vi "NML Signal Average.vi"() -> ()   [LabVIEW 2021]
doc: "Averages N cylces of input. Input is syncronized to a square wave output from DAC 1, DAC 0 is the drive of the given amplitude and duty cylce. Dac 1 should be connected to EXT Trigger, (make sure that DAC 1 has an external reference voltage of at least 1 V)\nScott Hannahs, FBNML, Jan 1992"
uses:
  <vilib>/_DAQmxBase/Internals/Properties/WriteProperties/RegenMode.ctl
  <vilib>/_DAQmxBase/Internals/DAQmxBase Create Channel (AO-Voltage-Basic).vi
  <vilib>/_DAQmxBase/Internals/DAQmxBase Timing (Sample Clock).vi
  <vilib>/_DAQmxBase/Internals/Properties/WriteProperties/Set_Write_RegenMode.vi
  <vilib>/_DAQmxBase/Internals/DAQmxBase Write (Analog 2D DBL NChan NSamp).vi
  <vilib>/_DAQmxBase/Internals/DAQmxBase Read (Analog 2D DBL NChan NSamp).vi
panel:
  out "Errors:":string
  out "?":dbl[](graph)
  out "Output Data":sgl[](array[numeric])=[0.032989502, 0.0625, 0.09112549, 0.12008667, 0.14807129, 0.17654419, 0.20431519, 0.23254395, 0.25964355, 0.2871704, 0.3139038, 0.34094238, 0.3671875, 0.39404297, 0.4197998, 0.44604492, 0.47161865, 0.49743652, 0.5225525, 0.5479126, 0.5722656, 0.59713745, 0.6213989, 0.64608765, 0.66989136, 0.6939392, 0.7173462, 0.74108887, 0.76416016, 0.78775024, 0.8104553, 0.8332825, 0.8556824, 0.8781738, 0.8999939, 0.9222717, 0.9437561, 0.9659729, 0.9867554, 1.0085449, 1.0292664, 1.0500183, 1.0709839, 1.0917358, 1.1118164, 1.1324463, 1.1521912, 1.1723633, 1.1917725, 1.2114258, 1.230835, 1.2502136, 1.2690735, 1.2883301, 1.3070068, 1.3257141, 1.3437195, 1.3625793, 1.3806763, 1.3986816, 1.4164429, 1.4342651, 1.4515991, 1.4693909, 1.4862976, 1.5037231, 1.5204773, 1.5375671, 1.5540771, 1.5710144, 1.5870056, 1.6036377, 1.6196594, 1.6356812, 1.6517029, 1.667572, 1.6828003, 1.6987, 1.7136536, 1.7294922, 1.7442322, 1.759552, 1.7741699, 1.7893372, 1.8037415, 1.8181763, 1.8328247, 1.8470154, 1.8611755, 1.8754272, 1.888977, 1.9031067, 1.9164734, 1.9305115, 1.9437256, 1.9572754, 1.9702454, 1.9837036, 1.9964905, 2.0097961, 2.0221863, 2.0352173, 2.047638, 2.0603638, 2.0722046, 2.0852966, 2.097107, 2.109314, 2.1211853, 2.1333008, 2.144867, 2.1571655, 2.1681519, 2.1801147, 2.190979, 2.2028503, 2.2136536, 2.2251282, 2.235962, 2.2472534, 2.2578125, 2.2688293, 2.2792969, 2.2900696, 2.3004456, 2.3112183, 2.3211975, 2.3319702, 2.3417053, 2.3520508, 2.3616333, 2.3719788, 2.3815613, 2.3916016, 2.4009705, 2.4106445, 2.4199219, 2.42984, 2.4389648, 2.4486694, 2.4572144, 2.4668884, 2.4756165, 2.4849548, 2.4935608, 2.502594, 2.5106506, 2.519806, 2.5283508, 2.5372314, 2.5454407, 2.5540466, 2.5621948, 2.5708008, 2.5786438, 2.5872192, 2.5947266, 2.6029663, 2.6105957, 2.618805, 2.6265564, 2.634552, 2.6419373, 2.6497803, 2.6569824, 2.6648865, 2.6722412, 2.679657, 2.686554, 2.694458, 2.7011414, 2.7087708, 2.715271, 2.7225342, 2.729309, 2.7364502, 2.7431946, 2.7503052, 2.7565002, 2.7634583, 2.7698975, 2.7767944, 2.782837, 2.7895813, 2.795929, 2.8024597, 2.8084412, 2.8148193, 2.8210754, 2.82724, 2.8332214, 2.8396606, 2.8454285, 2.8513184, 2.856842, 2.8631287, 2.868866, 2.8746338, 2.8800354, 2.8859863, 2.8912964, 2.8970642, 2.9022217, 2.9082336, 2.913147, 2.9189148, 2.9239807, 2.929596, 2.9346313, 2.940094, 2.9449158, 2.950409, 2.9551697, 2.9606323, 2.965332, 2.9704895, 2.9749756, 2.9799194, 2.9845886, 2.9897766, 2.9943848, 2.9996338, 3.003662, 3.008667, 3.0127563, 3.0178833, 3.0220642, 3.0269165, 3.0310059, 3.0357056, 3.0396423, 3.044403, 3.0485535, 3.0531006, 3.0569763, 3.061432, 3.065277, 3.0694275, 3.0734253, 3.0778198, 3.0814514, 3.085846, 3.0895996, 3.0937195, 3.09729, 3.10141, 3.1050415, 3.1092834, 3.1127625, 3.1166382, 3.1201172, 3.1239624, 3.127411, 3.131256, 3.1345215, 3.1383057, 3.142334, 3.1159668, 3.0895996, 3.0645142, 3.0388184, 3.0143738, 2.9890747, 2.9644775, 2.9400635, 2.9158325, 2.8914185, 2.8678894, 2.8439636, 2.8207703, 2.7972107, 2.774353, 2.7512207, 2.7288208, 2.705841, 2.684021, 2.6614075, 2.639923, 2.6178894, 2.596405, 2.574707, 2.5537415, 2.532318, 2.5117493, 2.4907227, 2.4706726, 2.4499512, 2.4298096, 2.4098816, 2.3901367, 2.3703003, 2.350708, 2.3310852, 2.3123474, 2.292633, 2.274109, 2.255127, 2.236969, 2.2182007, 2.2000122, 2.1818237, 2.1638489, 2.145996, 2.1282654, 2.1105347, 2.0935364, 2.0758057, 2.0591736, 2.041626, 2.025299, 2.0080566, 1.9917297, 1.9750977, 1.959259, 1.9427185, 1.927063, 1.910675, 1.8952637, 1.8792725, 1.8640747, 1.8486328, 1.8333435, 1.8180237, 1.8032837, 1.788269, 1.7736816, 1.7590637, 1.74469, 1.7299194, 1.716095, 1.7011719, 1.6877136, 1.6734314, 1.6602173, 1.6459961, 1.6327515, 1.6190186, 1.6058044, 1.5922852, 1.5796509, 1.5662842, 1.5537109, 1.5403748, 1.5280762, 1.5151672, 1.5027771, 1.4902039, 1.4781799, 1.4660339, 1.4541321, 1.4414673, 1.4299927, 1.4178162, 1.4064636, 1.3948059, 1.3835754, 1.3715515, 1.3607178, 1.348938, 1.3382568, 1.327179, 1.3163452, 1.3050232, 1.2947998, 1.283905, 1.2733765, 1.2626038, 1.2525635, 1.2420654, 1.231842, 1.2216797, 1.2118225, 1.2011414, 1.1916809, 1.1815186, 1.1719971, 1.1622009, 1.152832, 1.1428223, 1.1341858, 1.1242981, 1.1152039, 1.1057434, 1.0970459, 1.0876465, 1.07901, 1.0698547, 1.0611267, 1.052063, 1.0437622, 1.0348816, 1.0266418, 1.0179749, 1.0097351, 1.0010376, 0.9930725, 0.9847412, 0.97680664, 0.96832275, 0.96087646, 0.9525757, 0.9450073, 0.9370117, 0.92941284, 0.9214783, 0.9143677, 0.9063721, 0.89920044, 0.8913269, 0.8841553, 0.876709, 0.86987305, 0.86242676, 0.85549927, 0.84802246, 0.84140015, 0.83432007, 0.8274536, 0.8204651, 0.81411743, 0.80700684, 0.80062866, 0.79367065, 0.78744507, 0.7805481, 0.7746582, 0.76782227, 0.76171875, 0.7552185, 0.74902344, 0.7426758, 0.7367554, 0.7305298, 0.7247925, 0.7187195, 0.71273804, 0.70651245, 0.7012634, 0.6950989, 0.68969727, 0.68362427, 0.67837524, 0.67245483, 0.6670532, 0.6612549, 0.65625, 0.6502075, 0.64541626, 0.63986206, 0.6348877, 0.62924194, 0.6242676, 0.61898804, 0.6138916, 0.60839844, 0.6040039, 0.5985718, 0.5940552, 0.58877563, 0.58410645, 0.57891846, 0.57455444, 0.56954956, 0.5652771, 0.55999756, 0.55584717, 0.55078125, 0.54678345, 0.54177856, 0.53775024, 0.53289795, 0.5287781, 0.5241089, 0.5201416, 0.5155029, 0.5116272, 0.5070801, 0.5031738, 0.4984131, 0.49484253, 0.49053955, 0.48684692, 0.4822693, 0.47875977, 0.47436523, 0.47091675, 0.46676636, 0.46322632, 0.45880127, 0.45547485, 0.45135498, 0.44787598, 0.44384766, 0.44058228, 0.43643188, 0.433136, 0.4293213, 0.42593384, 0.42233276, 0.41903687, 0.41549683, 0.41204834, 0.40853882, 0.40551758, 0.4015503, 0.39855957, 0.39526367, 0.39227295, 0.3885498, 0.38589478, 0.38220215, 0.37924194, 0.37612915, 0.3730774, 0.36965942, 0.36679077, 0.3635559, 0.36080933, 0.3576355, 0.35488892, 0.35150146, 0.34902954, 0.34573364, 0.34317017, 0.3400879, 0.337677, 0.3345337, 0.3321228, 0.32907104, 0.32669067, 0.32357788, 0.32125854, 0.31814575, 0.31588745, 0.31292725, 0.31027222, 0.30789185, 0.30566406, 0.30273438, 0.30047607, 0.29779053, 0.29559326, 0.29284668, 0.29077148, 0.28796387, 0.28585815, 0.28311157, 0.28115845, 0.27841187, 0.27648926, 0.27386475, 0.2720337, 0.26931763, 0.26739502, 0.26474, 0.26293945, 0.2605896, 0.25872803, 0.25613403, 0.25424194, 0.25186157, 0.25012207, 0.24768066, 0.24609375, 0.24362183, 0.24209595, 0.23962402, 0.23788452, 0.23568726, 0.23413086, 0.23171997, 0.2303772, 0.22796631, 0.22647095, 0.22424316, 0.22265625, 0.22061157, 0.21884155, 0.21664429, 0.21530151, 0.21328735, 0.21166992, 0.20968628, 0.2083435, 0.20611572, 0.20483398, 0.20281982, 0.2013855, 0.1993103, 0.1979065, 0.19610596, 0.19473267, 0.1925354, 0.19174194, 0.18972778, 0.18832397, 0.18643188, 0.18518066, 0.18334961, 0.18209839, 0.18041992, 0.17919922, 0.17745972, 0.17602539, 0.1741333, 0.17324829, 0.17163086, 0.1706543, 0.16867065, 0.16744995, 0.16571045, 0.16473389, 0.16299438, 0.16210938, 0.16033936, 0.15924072, 0.15777588, 0.15667725, 0.15518188, 0.1541748, 0.15234375, 0.15164185, 0.14993286, 0.14907837, 0.14749146, 0.14627075, 0.14498901, 0.144104, 0.14260864, 0.14175415, 0.1402893, 0.1394043, 0.13790894, 0.13696289, 0.13562012, 0.13485718, 0.13342285, 0.13272095, 0.13110352, 0.13012695, 0.12890625, 0.12805176, 0.12658691, 0.1260376, 0.12463379, 0.12384033, 0.12258911, 0.121917725, 0.120513916, 0.11981201, 0.11846924, 0.11795044, 0.11654663, 0.115478516, 0.11444092, 0.11395264, 0.11260986, 0.112091064, 0.11077881, 0.11016846, 0.10882568, 0.10824585, 0.107055664, 0.1065979, 0.10543823, 0.10473633, 0.103637695, 0.10284424, 0.10168457, 0.10122681, 0.09994507, 0.09957886, 0.09829712, 0.09777832, 0.09674072, 0.09625244, 0.09515381, 0.09466553, 0.09371948, 0.09307861, 0.09210205, 0.09158325, 0.0904541, 0.0899353, 0.08898926, 0.08850098, 0.08734131, 0.0869751, 0.08581543, 0.08560181, 0.08441162, 0.08425903, 0.08303833, 0.08270264, 0.08178711, 0.08135986, 0.08013916, 0.07977295, 0.07891846, 0.078430176, 0.07763672, 0.07736206, 0.07626343, 0.0758667, 0.07495117, 0.07467651, 0.07366943, 0.07345581, 0.07260132, 0.07241821, 0.0713501, 0.07098389, 0.07009888, 0.06970215, 0.0687561, 0.06866455, 0.06793213, 0.0675354, 0.06655884, 0.066223145, 0.06536865, 0.06518555, 0.06442261, 0.06417847, 0.063201904, 0.062927246, 0.06210327, 0.061828613, 0.061035156, 0.060943604, 0.05999756, 0.05987549, 0.05899048, 0.05871582, 0.057891846, 0.05783081, 0.057128906, 0.056884766, 0.05609131, 0.05593872, 0.05505371, 0.054992676, 0.05407715, 0.054016113, 0.053222656, 0.05319214, 0.05230713, 0.052337646, 0.051483154, 0.051208496, 0.05050659, 0.050445557, 0.04989624, 0.04953003, 0.048736572, 0.048675537, 0.048065186, 0.04776001, 0.047088623, 0.04714966, 0.04626465, 0.046142578, 0.045440674, 0.045410156, 0.044921875, 0.044799805, 0.044067383, 0.04385376, 0.043273926, 0.043182373, 0.04244995, 0.042297363, 0.041809082, 0.041748047, 0.041046143, 0.041015625, 0.04043579, 0.040283203, 0.039520264, 0.039520264, 0.038848877, 0.038970947, 0.038116455, 0.038238525, 0.037475586, 0.03756714, 0.036834717, 0.036834717, 0.0362854, 0.036224365, 0.035491943, 0.035491943, 0.034942627, 0.034973145, 0.034362793, 0.034454346, 0.033935547, 0.033813477, 0.03302002, 0.033233643, 0.03265381, 0.032409668, 0.031829834, 0.03213501, 0.031555176, 0.031707764, 0.030914307, 0.030822754, 0.030395508, 0.030456543, 0.029754639, 0.030029297, 0.029266357, 0.029174805, 0.028778076, 0.028747559, 0.028289795, 0.028564453, 0.027832031, 0.027801514, 0.027191162, 0.027374268, 0.026733398, 0.026885986, 0.026275635, 0.026519775, 0.0256958, 0.025970459, 0.025543213, 0.025634766, 0.024780273, 0.02508545, 0.024597168, 0.024658203, 0.024017334, 0.024108887, 0.023590088, 0.023712158, 0.023071289, 0.023406982, 0.022857666, 0.022918701, 0.02243042, 0.022491455, 0.021942139, 0.021972656, 0.021575928, 0.02154541, 0.021118164, 0.021209717, 0.02053833, 0.020935059, 0.020446777, 0.02053833, 0.020080566, 0.020080566, 0.019592285, 0.019714355, 0.01928711, 0.019439697, 0.019012451, 0.019104004, 0.018676758, 0.018829346, 0.018218994, 0.018432617, 0.017822266, 0.017974854, 0.017578125, 0.0178833, 0.01727295, 0.017456055, 0.016906738, 0.016937256, 0.01663208, 0.016937256, 0.016326904, 0.01638794, 0.01586914, 0.015991211, 0.015594482, 0.015960693, 0.015655518, 0.015563965, 0.014923096, 0.0152282715, 0.01473999, 0.015167236, 0.014556885, 0.014678955, 0.014373779, 0.014404297, 0.013946533, 0.014007568, 0.01361084, 0.013885498, 0.013519287, 0.013641357, 0.013214111, 0.013458252, 0.012969971, 0.013305664, 0.012634277, 0.012878418, 0.012420654, 0.01260376, 0.012054443, 0.012359619, 0.0119018555, 0.012298584, 0.011810303, 0.0121154785, 0.01159668, 0.011627197, 0.011230469, 0.011444092, 0.011016846, 0.011291504, 0.010925293, 0.010955811, 0.0105896, 0.010955811, 0.010375977, 0.010772705, 0.0101623535, 0.010314941, 0.010101318, 0.010284424, 0.009918213, 0.009979248, 0.009490967, 0.009887695, 0.009399414, 0.009552002, 0.009155273, 0.009277344, 0.008911133, 0.009216309, 0.008758545, 0.008972168, 0.0087890625, 0.00881958, 0.008575439, 0.00869751, 0.008270264, 0.008514404, 0.008056641, 0.008361816, 0.007965088, 0.0079956055, 0.007843018, 0.0079956055, 0.007598877, 0.007873535, 0.007507324, 0.0077819824, 0.0071411133, 0.007385254, 0.0071105957, 0.007446289, 0.006958008, 0.0072631836, 0.00680542, 0.007019043, 0.0065307617, 0.0068359375, 0.0064697266, 0.006866455, 0.006500244, 0.0067749023, 0.006286621, 0.006439209, 0.006011963, 0.0062561035, 0.0059509277, 0.0063476562, 0.0058898926, 0.006072998, 0.0056152344, 0.005706787, 0.005432129, 0.005645752, 0.0054626465, 0.00579834, 0.0053710938, 0.005584717, 0.005065918, 0.0053710938, 0.0050354004, 0.0053100586, 0.0048217773, 0.005126953, 0.004760742, 0.004852295, 0.004425049, 0.0048217773, 0.0046691895, 0.004760742, 0.0045776367, 0.004760742, 0.004272461, 0.004547119, 0.0043029785, 0.004486084, 0.004119873, 0.004486084, 0.003967285, 0.004180908, 0.003753662, 0.004058838, 0.0038452148, 0.003967285, 0.003692627, 0.004058838, 0.0035705566, 0.0038452148, 0.0034484863, 0.0038146973, 0.0033874512, 0.0037841797, 0.003326416, 0.0035705566, 0.0030822754, 0.0028686523] format="%.5f"
  out "Drive Channel #0":dbl[](graph)
  in  "Comments":string="This data's for you."
  in  "User Name":string="Conan the SCIENTIST"
  in  "File":string="Test"
  out "File Name":string
  in  "Amplitude":dbl=10.0 format="%.2f"
  in  "Offset":dbl format="%.2f"
  in  "# of Samples":i32=1024
  in  "Period (msec)":sgl=500.0 min=0.01 max=1000000 format="%.2f"
  in  "Channel #":i16(slide) min=0 max=7 step=1 scale=0.0..7.0
  in  "Gain":i16(slide) min=0 max=3 step=1 scale=0.0..3.0
  in  "Duty Cycle":dbl=0.5 min=0.009999999776482582 max=0.9899999499320984 format="%.2f"
  in  "Cycles to Average":i32=10 min=1 max=100000
  out "Frequcncy (Hz)":sgl=1.9970603 min=0.0009999999 max=100000 format="%.4f"
  # "Time (msec)"
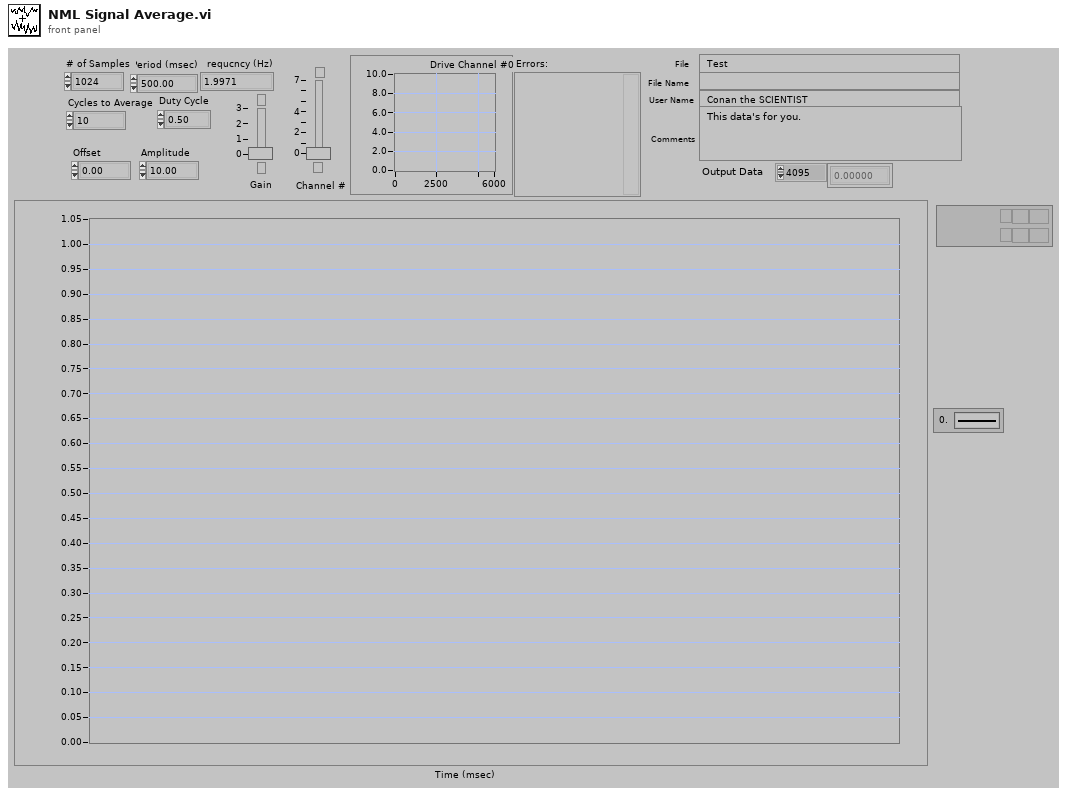
[diagram p1: front panel]
types:
  T1 = typedef "RegenMode.ctl" = i32
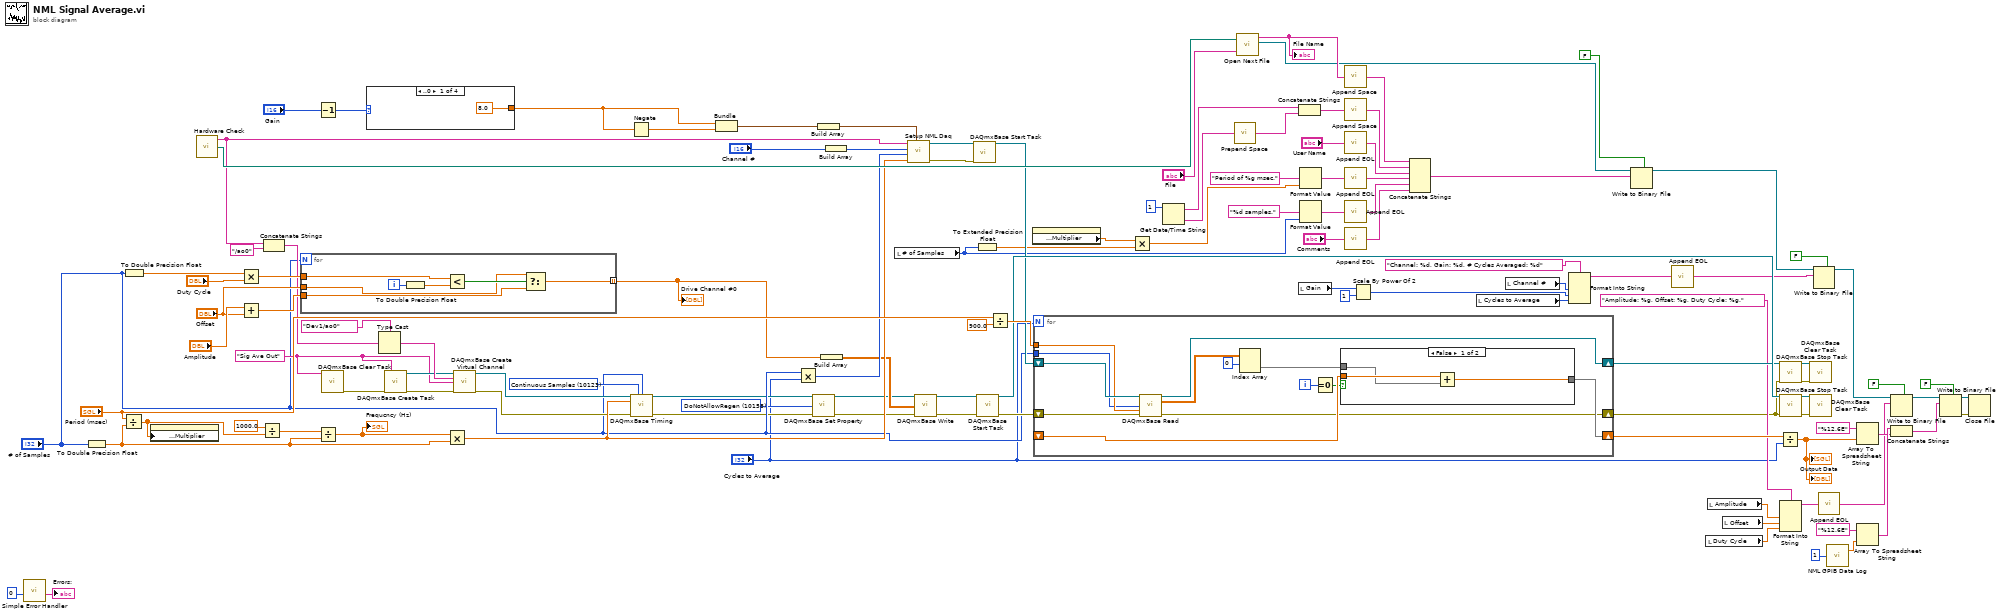
[diagram p0: block diagram]
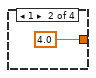
[diagram p3: hidden frame]
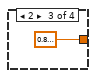
[diagram p4: hidden frame]
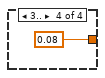
[diagram p5: hidden frame]
diagram:
  w46 = T1 10158 items=["AllowRegen"=10097, "DoNotAllowRegen"=10158] ("RegenMode")
  w81 = 10123 items=["Finite Samples"=10178, "Continuous Samples"=10123, "Hardware Timed Single Point"=12522] ("sample mode")
  w57 = "Sig Ave Out"
  n1 = call <vilib>:"Simple Error Handler.vi"("type of dialog (OK msg:1)"=0) -> ("source out"=→"Errors:":string)  [unwired: 4 in, 4 out]
  n2 = To Double Precision Float(number="# of Samples") -> (double precision float=w114:dbl)
  n3 = Divide(x="Period (msec)", y=w114) -> (x/y=w112:dbl)
  n4 = To Double Precision Float(number="# of Samples") -> (double precision float=w55:dbl)
  n5 = property class="WFGraph (strict)"("X Scale.Offset and Multiplier:Multiplier"=w112) -> ()  [unwired: 2 in, 2 out]
  n6 = call "Hardware Check.vi"() -> ("Data Acq Device"=w97:string, "Data Directory Path"=w109:path)  [unwired: 1 in, 1 out]
  n7 = Multiply(x=w55, y="Duty Cycle") -> (x*y=w91:dbl)
  n8 = Add(x="Amplitude", y="Offset") -> (x+y=w89:dbl)
  n9 = Divide(x=sgl 1000.0, y=w112) -> (x/y=w117:dbl)
  n10 = Concatenate Strings(w97, "/ao0" ("string")) -> (w84:string)
  n11 = for {
    N: "# of Samples" -> [_]
    tunnel: "Offset" -> [w122]
    tunnel: w89 -> [w121]
    tunnel: w91 -> [w124]
    tunnel: [w120] -> w80 mode=indexing
    i -> [w125]
    n12 = To Double Precision Float(number=w125) -> (double precision float=w119:dbl)
    n13 = Less?(x=w124, y=w119) -> (x < y?=w123:bool)
    n14 = Select(t=w122, s=w123, f=w121) -> (s? t:f=w120:dbl)
  }
  "Drive Channel #0" <- w80
  n15 = Decrement(x="Gain") -> (x-1=w105:i16)
  n16 = Divide(x=w117, y=w114) -> (x/y=w115:dbl)
  "Frequcncy (Hz)" <- w115
  n17 = call <vilib>:"DAQmxBase Clear Task.vi"("task in"=w57) -> ("error out"=w60:errorcluster)  [unwired: 14 in]
  n18 = case shown="..0" w105 {
    tunnel: [8.0 sgl 4.0 sgl 0.8 0.08] -> w103
    frame ..0 {
    }
    frame 1 {
    }
    frame 2 {
    }
    frame 3.. {
    }
  }
  n19 = Type Cast(type=tag "Dev1/ao0" ("physical channels"), x=w84) -> (*(type *) &x=w86:tag)
  n20 = call <vilib>:"DAQmxBase Create Task.vi"("new task name"=w57, "error in"=w60) -> ("task out"=w58:refnum<k21>, "error out"=w59:errorcluster)  [unwired: 12 in]
  n21 = Multiply(x=w115, y=w114) -> (x*y=w98:dbl)
  n22 = call-poly <vilib>:"DAQmxBase Create Virtual Channel.vi"("task in"=w58, "physical channels"=w86, "name to assign"=w57, "error in"=w59) -> ("task out"=w83:refnum<k21>, "error out"=w82:errorcluster)  [unwired: 10 in]
  n23 = Negate(x=w103) -> (-x=w104:dbl)
  n24 = call-poly <vilib>:"DAQmxBase Timing.vi"("task/channels in"=w83, "sample mode"=w81, "samples per channel"="# of Samples", "rate"=w98, "error in"=w82) -> ("task out"=w48:refnum<k21>, "error out"=w47:errorcluster)  [unwired: 9 in]
  n25 = Bundle(w103, w104) -> (w101:cluster{dbl, dbl})  [unwired: 1 in]
  n26 = Multiply(x="# of Samples", y="Cycles to Average") -> (x*y=w96:i32)
  n27 = call-poly <vilib>:"DAQmxBase Set Property.vi"("task/channels in"=w48, "RegenMode"=w46, "error in"=w47) -> ("task out"=w49:refnum<k21>, "error out"=w50:errorcluster)  [unwired: 11 in]
  n28 = Build Array(w101) -> (w100:cluster{dbl, dbl}[])
  n29 = Build Array(w80) -> (w56:dbl[][])
  n30 = Build Array("Channel #") -> (w99:i16[])
  n31 = local read "# of Samples"() -> (w22:i32)
  n32 = call "Setup NML Daq.vi"("Input Limits"=w100, "rate"=w98, "number of samples per channel"=w96, "channels (0)"=w99, "Data Acq Device"=w97) -> ("error out"=w94:errorcluster, "task out"=w95:refnum<k21>)  [unwired: 5 in]
  n33 = call-poly <vilib>:"DAQmxBase Write.vi"("task/channels in"=w49, "data"=w56, "error in"=w50) -> ("task out"=w78:refnum<k21>, "error out"=w79:errorcluster)  [unwired: 10 in, 1 out]
  n34 = call <vilib>:"DAQmxBase Start Task.vi"("task/channels in"=w95, "error in"=w94) -> ("task out"=w93:refnum<k21>)  [unwired: 12 in, 1 out]
  n35 = To Extended Precision Float(1:w22) -> (0:w25:ext)
  n36 = call <vilib>:"DAQmxBase Start Task.vi"("task/channels in"=w78, "error in"=w79) -> ("task out"=w107:refnum<k21>, "error out"=w110:errorcluster)  [unwired: 12 in]
  n37 = Divide(x="Period (msec)", y=sgl 900.0) -> (x/y=w111:sgl)
  n38 = property class="WFGraph (strict)"() -> ("X Scale.Offset and Multiplier:Multiplier"=w23:dbl)  [unwired: 2 in, 2 out]
  n39 = for {
    N: "Cycles to Average" -> [_]
    shift-right: [w142] -> w77
    shift-left: _ -> [w141]
    tunnel: "# of Samples" -> [w132]
    shift-right: [w134] -> w3
    shift-left: w110 -> [w135]
    tunnel: w111 -> [w133]
    shift-right: [w131] -> w53
    shift-left: w93 -> [w140]
    i -> [w139]
    n40 = call-poly <vilib>:"DAQmxBase Read.vi"("task/channels in"=w140, "number of samples per channel"=w132, "timeout"=w133, "error in"=w135) -> ("task out"=w131:refnum<k21>, "data"=w137:dbl[][], "error out"=w134:errorcluster)  [unwired: 9 in]
    n41 = Index Array(array=w137, index (row)=0) -> (element=w136:dbl[])  [unwired: 1 in]
    n42 = Equal To 0?(x=w139) -> (x = 0?=w138:bool)
    n43 = case shown="False" w138 {
      tunnel: w141 -> [w145 _]
      tunnel: [w144 w146] -> w142
      tunnel: w136 -> [w143 w146]
      frame False {
        n44 = Add(x=w145, y=w143) -> (x+y=w144:dbl[])
      }
      frame True {
      }
    }
  }
  n45 = Multiply(x=w23, y=w25) -> (x*y=w26:ext)
  n46 = Get Date/Time String(date format (0)=1) -> (date string=w32:string, time string=w30:string)  [unwired: 2 in]
  n47 = call "Prepend Space.vi"("Input String"=w30) -> ("Space + Input String"=w31:string)
  n48 = call "Open Next File.vi"("Input File Pattern"="File", "Dir Path"=w109) -> ("File Ref Num"=w68:refnum<file>, "Output File Name"=w73:string)  [unwired: 1 in, 2 out]
  "File Name" <- w73
  n49 = Concatenate Strings(w32, w31) -> (w33:string)
  n50 = local read "Gain"() -> (w14:i16)
  n51 = Format Value(format string="Period of %g msec.", value (0)=w26) -> (output string=w40:string)  [unwired: 1 in]
  n52 = Format Value(format string="%d samples.", value (0)=w22) -> (output string=w41:string)  [unwired: 1 in]
  n53 = call "Append Space.vi"("INPUT STRING"=w73) -> ("OUTPUT STRING (PLUS [SPACE])"=w39:string)
  n54 = call "Append Space.vi"("INPUT STRING"=w33) -> ("OUTPUT STRING (PLUS [SPACE])"=w38:string)
  n55 = call "Append EOL.vi"("INPUT STRING"="User Name") -> ("OUTPUT STRING (PLUS End of Line)"=w37:string)
  n56 = call "Append EOL.vi"("INPUT STRING"=w40) -> ("OUTPUT STRING (PLUS End of Line)"=w36:string)
  n57 = call "Append EOL.vi"("INPUT STRING"=w41) -> ("OUTPUT STRING (PLUS End of Line)"=w35:string)
  n58 = call "Append EOL.vi"("INPUT STRING"="Comments") -> ("OUTPUT STRING (PLUS End of Line)"=w34:string)
  n59 = Scale By Power Of 2(n=w14, x=1) -> (x*2^n=w16:i32)
  n60 = Concatenate Strings(w39, w38, w37, w36, w35, w34) -> (w24:string)
  n61 = local read "Cycles to Average"() -> (w15:i32)
  n62 = local read "Channel #"() -> (w13:i16)
  n63 = Format Into String(format string="Channel: %d, Gain: %d, # Cycles Averaged: %d", w13, w16, w15) -> (resulting string=w18:string)  [unwired: 2 in, 1 out]
  n64 = Write to Binary File(file (use dialog)=w68, data=w24, 5:FALSE ("prepend array or string size? (T)")) -> (refnum out=w45:refnum<file>)  [unwired: 3 in, 2 out]
  n65 = call "Append EOL.vi"("INPUT STRING"=w18) -> ("OUTPUT STRING (PLUS End of Line)"=w20:string)
  n66 = local read "Duty Cycle"() -> (w8:dbl)
  n67 = local read "Amplitude"() -> (w7:dbl)
  n68 = local read "Offset"() -> (w6:dbl)
  n69 = call <vilib>:"DAQmxBase Stop Task.vi"("task/channels in"=w53, "error in"=w3) -> ("task out"=w52:refnum<k21>, "error out"=w2:errorcluster)  [unwired: 12 in]
  n70 = call <vilib>:"DAQmxBase Stop Task.vi"("task/channels in"=w107, "error in"=w3) -> ("task out"=w54:refnum<k21>, "error out"=w4:errorcluster)  [unwired: 12 in]
  n71 = Divide(x=w77, y="Cycles to Average") -> (x/y=w108:dbl[])
  "Output Data" <- w108
  "?" <- w108
  n72 = Format Into String(format string="Amplitude: %g, Offset: %g, Duty Cycle: %g.", w7, w6, w8) -> (resulting string=w9:string)  [unwired: 2 in, 1 out]
  n73 = call <vilib>:"DAQmxBase Clear Task.vi"("task in"=w52, "error in"=w2) -> ()  [unwired: 13 in, 1 out]
  n74 = call <vilib>:"DAQmxBase Clear Task.vi"("task in"=w54, "error in"=w4) -> ()  [unwired: 13 in, 1 out]
  n75 = Write to Binary File(file (use dialog)=w45, data=w20, 5:FALSE ("prepend array or string size? (T)")) -> (refnum out=w44:refnum<file>)  [unwired: 3 in, 2 out]
  n76 = call "Append EOL.vi"("INPUT STRING"=w9) -> ("OUTPUT STRING (PLUS End of Line)"=w11:string)
  n77 = call "NML GPIB Data Log.vi"("Point #"=1) -> ("GPIB Data"=w67:dbl[])  [unwired: 1 out]
  n78 = Array To Spreadsheet String(array=w108, 3:"%12.6E") -> (spreadsheet string=w63:string)  [unwired: 1 in]
  n79 = Array To Spreadsheet String(array=w67, 3:"%12.6E") -> (spreadsheet string=w64:string)  [unwired: 1 in]
  n80 = Write to Binary File(file (use dialog)=w44, data=w11, 5:FALSE ("prepend array or string size? (T)")) -> (refnum out=w69:refnum<file>)  [unwired: 3 in, 2 out]
  n81 = Concatenate Strings(w64, w63) -> (w62:string)
  n82 = Write to Binary File(file (use dialog)=w69, data=w62, 5:FALSE ("prepend array or string size? (T)")) -> (refnum out=w71:refnum<file>, error out=w70:errorcluster)  [unwired: 3 in, 1 out]
  n83 = Close File(refnum=w71, error in=w70) -> ()  [unwired: 2 out]
